vi "New Assert Message.vi"(8 "error in (no error)":errorcluster, 10 "Assert Message":string, 11 "Main Display in":refnum<class "Main Display.lvclass">) -> (0 "error out":errorcluster, 3 "Main Display out":refnum<class "Main Display.lvclass">)   [LabVIEW 2016, in "Assert API Components.lvlib" / "Assert Display.lvlib" / "Main Display.lvlib" / "Main Display.lvclass"]
uses:
  Main Display.lvclass
  Assert API Components/Message Data.ctl
  Assert API Components/Failure Actions.ctl
  Assert API Components/VI References.ctl
  Main Display.lvclass/Main Display.ctl
  <resource>/AFDebug/Localized Strings.vi
  <resource>/AFDebug/Get Clone Name.vi
  <resource>/AFDebug/Actor Registry.vi
  <resource>/AFDebug/TDM Registry.vi
  Display Configurations/Base Display Configuration.lvclass
  Assert API Components/Assert API Components.lvlib
  <resource>/AFDebug/AF Debug.lvlib
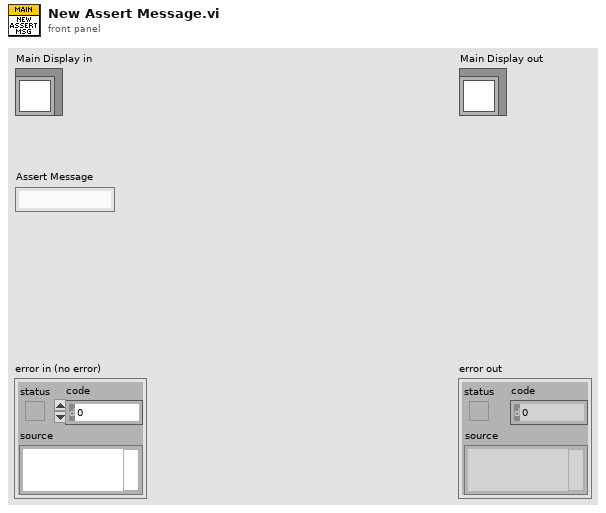
[diagram p1: front panel]
types:
  T1 = typedef "Assert API Components.lvlib/Message Data.ctl" = cluster{"Data Value":variant, "Last Update":timestamp, "Comment":string, "Evaluation String":string, "Status":bool, "Assert Name":string, "Failure Action":T2, "Assert VI Name":string, "Calling VI Name":string, "Assert VI UID":i32, "Top Level VI Name":string, "VI References":T3, "Assert Build Timestamp":timestamp, "Assert Builder User Name":string, "Data Type":string, "IP Address":string}
  T2 = typedef "Assert API Components.lvlib/Failure Actions.ctl" = enum16{"None", "Log To File", "Pause Execution", "Abort Execution"}
  T3 = typedef "Assert API Components.lvlib/VI References.ctl" = cluster{"Calling VI Ref":refnum<vi>, "Assert VI Ref":refnum<vi>}
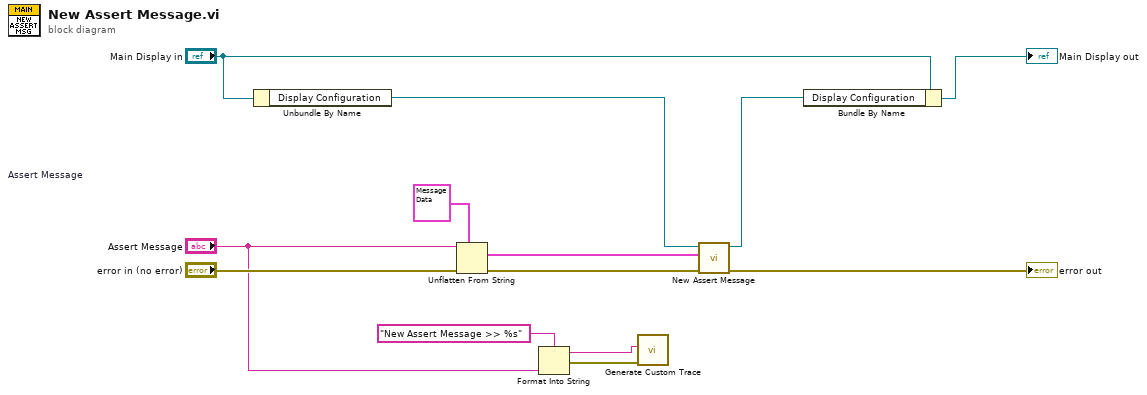
[diagram p0: block diagram]
diagram:
  w11 = T1 {"Data Value"=variant, "Last Update"=timestamp(0 s since 1904-01-01), "Comment"="", "Evaluation String"="", "Status"=FALSE, "Assert Name"="", "Failure Action"=enum."None", "Assert VI Name"="", "Calling VI Name"="", "Assert VI UID"=0, "Top Level VI Name"="", "VI References"={"Calling VI Ref"=refnum, "Assert VI Ref"=refnum}, "Assert Build Timestamp"=timestamp(0 s since 1904-01-01), "Assert Builder User Name"="", "Data Type"="", "IP Address"=""}  # Assert Message
  n1 = Unbundle By Name("Main Display in") -> ("Display Configuration"=w10:refnum<class "Base Display Configuration.lvclass">)
  n2 = Unflatten From String(type=w11, binary string="Assert Message", error in (no error)="error in (no error)") -> (value=w5:T1, error out=w12:errorcluster)  [unwired: 2 in, 1 out]
  n3 = Format Into String(format string="New Assert Message >> %s", "Assert Message") -> (resulting string=w2:string, error out=w1:errorcluster)  [unwired: 2 in]
  n4 = call <resource>:"Generate Custom Trace.vi"("error in (no error)"=w1, "Custom Action"=w2) -> ()  [unwired: 10 in]
  n5 = call-dynamic "New Assert Message.vi"("error in (no error)"=w12, "Assert Message"=w5, "Base Display Configuration in"=w10) -> ("error out"=→"error out":errorcluster, "Base Display Configuration out"=w9:refnum<class "Base Display Configuration.lvclass">)  [unwired: 7 in]
  n6 = Bundle By Name(cluster="Main Display in", "Display Configuration"=w9) -> (→"Main Display out":refnum<class "Main Display.lvclass">)
